vi "Write Waveform to Log File Instance.vi"(6 "Data":dbl[](array[numeric]), 7 "Segmented Log Waveform Meta Data":T1, 8 "error in (no error)":errorcluster, 9 "Channel Name in":string, 11 "Segmented Log in":refnum<class "Segmented Log.lvclass">) -> (0 "error out":errorcluster, 1 "File Segmented":bool, 2 "Log Active":bool, 3 "Segmented Log out":refnum<class "Segmented Log.lvclass">)   [LabVIEW 2012, in "Waveform Data Logger Engine.lvlib" / "Segmented Log.lvclass"]
doc: "Writes data to a log file instance. If the segmented log is still active, ensures a valid file instance is open before logging data. After each write operation, checks if the current file instance has surpassed any limits and needs to be closed."
uses:
  Segmented Log.lvclass
  Segmented Log Waveform Meta Data.ctl
  Segmented Log.lvclass/Segmented Log.ctl
  Shared/Classes/Log File Specifications/Log File Specification/Log File Specification.lvclass/Log File Specification.ctl
  Shared/Classes/Log File Specifications/Waveform TDMS Log File Specification/Waveform TDMS Log File Specification.lvclass
  Shared/Classes/Log File Specifications/Waveform TDMS Log File Specification/Waveform TDMS Log File Specification.lvclass/Waveform TDMS Log File Specification.ctl
  Log Files/Log File/Log File.lvclass/Log File.ctl
  Log Files/TDMS Log File/TDMS Log File.lvclass
  Log Files/TDMS Log File/TDMS Log File.lvclass/TDMS Log File.ctl
  Close Log File Instance.vi
  Open Log File Instance.vi
  On Segmented Log Complete.vi
  On File Close.vi
  Shared/Classes/Log File Specifications/Log File Specification/Open Log File.vi
  Shared/Classes/Log File Specifications/Log File Specification/Set Path Tag.vi
  On File Open.vi
  Shared/Classes/Log File Specifications/Log File Specification/Set Filename Offset.vi
  Shared/Classes/Log File Specifications/Log File Specification/Build File Path.vi
  Shared/Classes/Log File Specifications/Log File Specification/Resolve File Conflicts.vi
  Shared/Classes/Log File Specifications/Log File Specification/Initialize Log File.vi
  <vilib>/Utility/libraryn.llb/Check if File or Folder Exists.vi
  <vilib>/Utility/error.llb/Error Cluster From Error Code.vi
  <vilib>/Utility/libraryn.llb/Get File Extension.vi
  <vilib>/Utility/libraryn.llb/Create Directory Recursive.vi
  Segment Log File.vi
  Log Files/Log File/Close Log File.vi
  Make File Read-Only.vi
  Log Files/Log File/Log File.lvclass
  Shared/Classes/Log File Specifications/Log File Specification/Log File Specification.lvclass
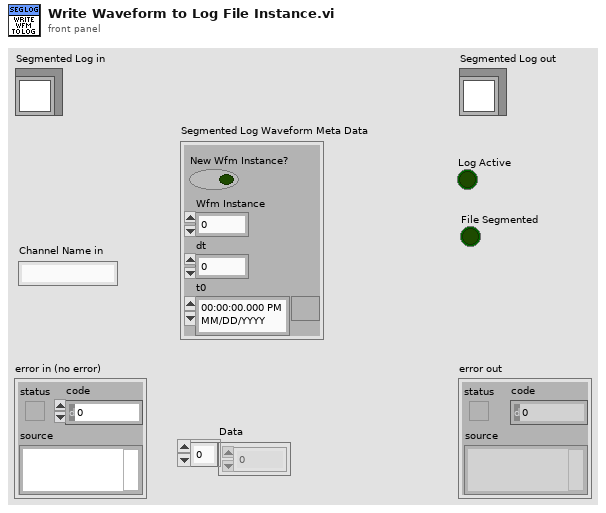
[diagram p1: front panel]
types:
  T1 = typedef "Waveform Data Logger Engine.lvlib/Segmented Log.lvclass/Segmented Log Waveform Meta Data.ctl" = cluster{"New Wfm Instance?":bool, "Wfm Instance":i32, "dt":dbl, "t0":timestamp}
  T2 = typedef "Waveform Data Logger Shared.lvlib/Log File Specification.lvclass/Log Specification Type.ctl" = enum16{"Default", "TDMS", "Text", "Waveform TDMS"}
  T3 = typedef "Waveform Data Logger Engine.lvlib/Log File.lvclass/Log File Type.ctl" = enum16{"Default", "TDMS", "Text"}
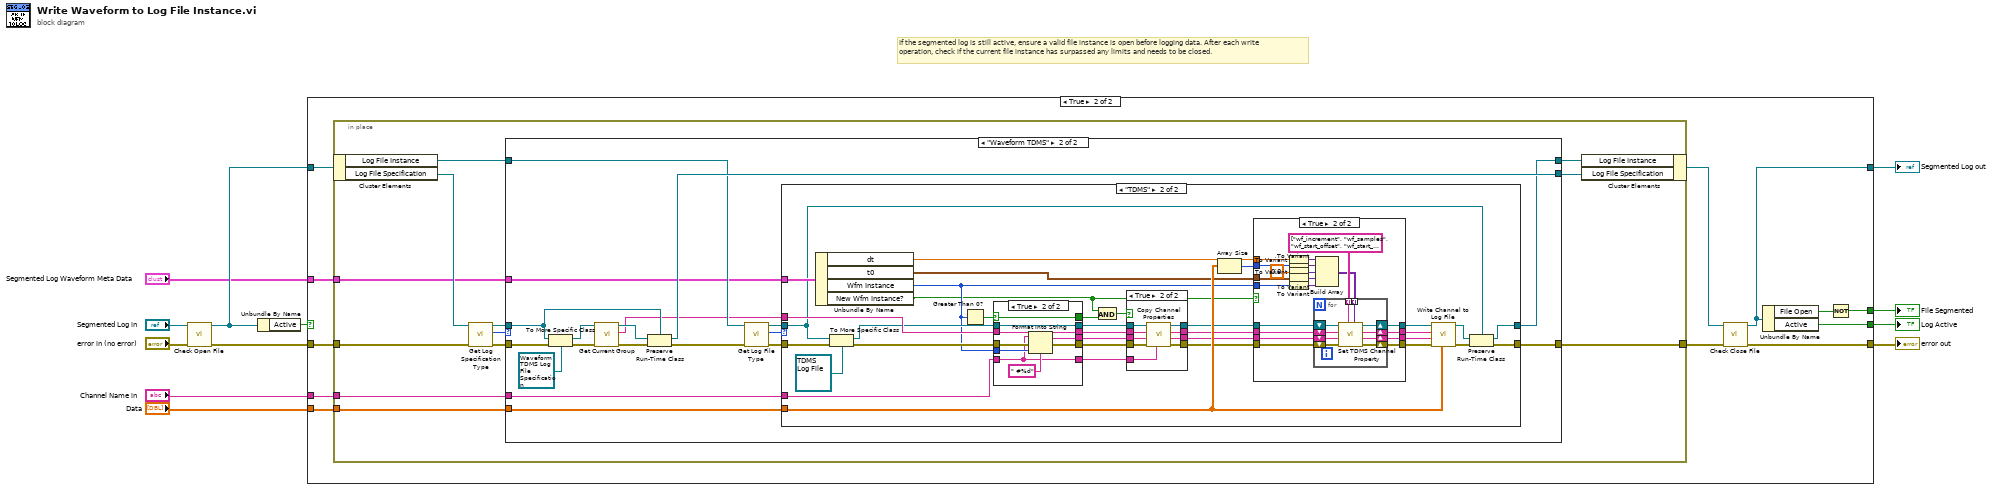
[diagram p0: block diagram]
diagram:
  # "If the segmented log is still active, ensure a valid file instance is open before logging data. After each write operation, check if the current file instance has surpassed any limits and needs to be closed."
  n1 = call "Check Open File.vi"("error in (no error)"="error in (no error)", "Segmented Log in"="Segmented Log in") -> ("error out"=w7:errorcluster, "Segmented Log out"=w6:refnum<class "Segmented Log.lvclass">)  [unwired: 8 in]
  n2 = Unbundle By Name(w6) -> ("Active"=w5:bool)
  n3 = case shown="True" w5 {
    selector: w5 -> [w14 _]
    tunnel: w7 -> [w15 w24]
    tunnel: "Channel Name in" -> [_ w23]
    tunnel: "Data" -> [_ w27]
    tunnel: [w13 w21] -> w10
    tunnel: [w15 w25] -> w11
    tunnel: w6 -> [w13 w22]
    tunnel: [w14 w20] -> w8
    tunnel: "Segmented Log Waveform Meta Data" -> [_ w19]
    tunnel: [_ w16] -> w1
    frame False {
      # "This segmented logging configuration is no longer active."
    }
    frame True {
      n4 = in-place {
        in-place-border: w27 -> [w39]
        in-place-border: [w38] -> w26
        in-place-border: w24 -> [w34]
        in-place-border: w23 -> [w37]
        in-place-border: w19 -> [w29]
        n5 = in-place-cluster #1(w22) -> ("Log File Instance"=w28:refnum<class "Log File.lvclass">, "Log File Specification"=w32:refnum<class "Log File Specification.lvclass">)
        n6 = call "Get Log Specification Type.vi"("error in (no error)"=w34, "Log File Specification in"=w32) -> ("error out"=w33:errorcluster, "Log Specification Type"=w30:T2, "Log File Specification out"=w31:refnum<class "Log File Specification.lvclass">)  [unwired: 7 in]
        n7 = case shown="\"Waveform TDMS\"" w30 {
          tunnel: w39 -> [_ w61]
          tunnel: [w42 w47] -> w38
          tunnel: w37 -> [_ w60]
          tunnel: w28 -> [w41 w51]
          tunnel: [w41 w46] -> w36
          tunnel: [w40 w54] -> w35
          tunnel: w33 -> [w42 w53]
          tunnel: w31 -> [w40 w52]
          tunnel: w29 -> [_ w43]
          frame Default {
            # "TODO-LATER: Throw Error"
          }
          frame "Waveform TDMS" {
            n8 = To More Specific Class(target class=refnum<class "Waveform TDMS Log File Specification.lvclass"> refnum ("Waveform Data Logger Engine.lvlib:Waveform TDMS Log File Specification.lvclass"), reference=w52, error in=w53) -> (specific class reference=w57:refnum<class "Waveform TDMS Log File Specification.lvclass">, error out=w58:errorcluster)
            n9 = call "Get Current Group.vi"("error in (no error)"=w58, "Waveform TDMS Log File Specification in"=w57) -> ("error out"=w56:errorcluster, "Current Group"=w44:string, "Waveform TDMS Log File Specification out"=w55:refnum<class "Waveform TDMS Log File Specification.lvclass">)  [unwired: 7 in]
            n10 = Preserve Run-Time Class(object in=w55, error in=w56, 2:w52) -> (object out=w54:refnum<class "Log File Specification.lvclass">, error out=w50:errorcluster)
            n11 = call "Get Log File Type.vi"("error in (no error)"=w50, "Log File in"=w51) -> ("error out"=w48:errorcluster, "Log File Type"=w45:T3, "Log File out"=w49:refnum<class "Log File.lvclass">)  [unwired: 7 in]
            n12 = case shown="\"TDMS\"" w45 {
              tunnel: w61 -> [_ w82]
              tunnel: w60 -> [_ w77]
              tunnel: w49 -> [w62 w83]
              tunnel: w48 -> [w63 w93]
              tunnel: [w63 w95] -> w47
              tunnel: [w62 w94] -> w46
              tunnel: w44 -> [_ w89]
              tunnel: w43 -> [_ w91]
              frame "Default", Default {
                # "TODO-LATER: Throw error"
                # ": Throw Error"
              }
              frame "TDMS" {
                n13 = Unbundle By Name(w91) -> ("dt"=w87:dbl, "t0"=w64:timestamp, "Wfm Instance"=w80:i32, "New Wfm Instance?"=w65:bool)
                n14 = To More Specific Class(target class=refnum<class "TDMS Log File.lvclass"> refnum ("TDMS Log File in"), reference=w83, error in=w93) -> (specific class reference=w88:refnum<class "TDMS Log File.lvclass">, error out=w90:errorcluster)
                n15 = Greater Than 0?(x=w80) -> (x > 0?=w78:bool)
                n16 = case shown="True" w78 {
                  selector: w78 -> [w145 w150]
                  tunnel: w90 -> [w147 w156]
                  tunnel: w89 -> [w148 w154]
                  tunnel: w77 -> [w146 w151]
                  tunnel: w80 -> [_ w158]
                  tunnel: [w148 w154] -> w72
                  tunnel: [w146 w152] -> w71
                  tunnel: [w147 w153] -> w70
                  tunnel: [w149 w155] -> w73
                  tunnel: w88 -> [w149 w155]
                  tunnel: [w146 w151] -> w76
                  tunnel: [w145 w150] -> w75
                  frame False {
                  }
                  frame True {
                    n17 = Format Into String(format string=" #%d", initial string=w151, error in=w156, w158) -> (resulting string=w152:string, error out=w153:errorcluster)
                  }
                }
                n18 = And(x=w65, y=w75) -> (x .and. y?=w74:bool)
                n19 = case shown="True" w74 {
                  tunnel: w76 -> [_ w110]
                  tunnel: w73 -> [w101 w109]
                  tunnel: w72 -> [w100 w108]
                  tunnel: w71 -> [w99 w107]
                  tunnel: w70 -> [w98 w106]
                  tunnel: [w101 w105] -> w69
                  tunnel: [w100 w104] -> w68
                  tunnel: [w99 w103] -> w67
                  tunnel: [w98 w102] -> w66
                  frame False {
                  }
                  frame True {
                    n20 = call "Copy Channel Properties.vi"("Base Channel"=w110, "error in (no error)"=w106, "New Channel in"=w107, "Group Name in"=w108, "TDMS Log File in"=w109) -> ("error out"=w102:errorcluster, "New Channel out"=w103:string, "Group Name out"=w104:string, "TDMS Log File out"=w105:refnum<class "TDMS Log File.lvclass">)  [unwired: 3 in]
                  }
                }
                n21 = Array Size(array=w82) -> (size(s)=w81:i32)
                n22 = case shown="True" w65 {
                  tunnel: w66 -> [w111 w115]
                  tunnel: w67 -> [w112 w116]
                  tunnel: w68 -> [w113 w117]
                  tunnel: w69 -> [w114 w118]
                  tunnel: w87 -> [_ w120]
                  tunnel: w64 -> [_ w133]
                  tunnel: [w114 w126] -> w86
                  tunnel: [w113 w125] -> w85
                  tunnel: [w112 w124] -> w79
                  tunnel: [w111 w123] -> w84
                  tunnel: w81 -> [_ w122]
                  tunnel: w80 -> [_ w119]
                  frame False {
                  }
                  frame True {
                    n23 = To Variant(anything=w120) -> (Variant=w130:variant)
                    n24 = To Variant(anything=w122) -> (Variant=w128:variant)
                    n25 = To Variant(anything=0.0) -> (Variant=w131:variant)
                    n26 = To Variant(anything=w133) -> (Variant=w129:variant)
                    n27 = To Variant(anything=w119) -> (Variant=w121:variant)
                    n28 = Build Array(w130, w128, w131, w129, w121) -> (w127:variant[])
                    n29 = for {
                      shift-right: [w143] -> w123
                      shift-left: w115 -> [w144]
                      shift-right: [w139] -> w124
                      shift-left: w116 -> [w142]
                      shift-right: [w140] -> w125
                      shift-left: w117 -> [w141]
                      shift-right: [w137] -> w126
                      shift-left: w118 -> [w138]
                      tunnel: string[] ["wf_increment", "wf_samples", "wf_start_offset", "wf_start_time", "Waveform Instance"] ("property names") -> [w136] mode=indexing
                      tunnel: w127 -> [w135] mode=indexing
                      n30 = call "Set TDMS Channel Property.vi"("Property Value"=w135, "Property Name"=w136, "error in (no error)"=w144, "Channel Name in"=w142, "Group Name in"=w141, "TDMS Log File in"=w138) -> ("error out"=w143:errorcluster, "Channel Name out"=w139:string, "Group Name out"=w140:string, "TDMS Log File out"=w137:refnum<class "TDMS Log File.lvclass">)  [unwired: 2 in]
                    }
                  }
                }
                n31 = call "Write Channel to Log File.vi"("Data"=w82, "error in (no error)"=w84, "Channel Name in"=w79, "Group Name in"=w85, "Log File in"=w86) -> ("error out"=w97:errorcluster, "Log File out"=w96:refnum<class "TDMS Log File.lvclass">)  [unwired: 5 in]
                n32 = Preserve Run-Time Class(object in=w96, error in=w97, 2:w83) -> (object out=w94:refnum<class "Log File.lvclass">, error out=w95:errorcluster)
              }
            }
          }
        }
        n33 = in-place-cluster #1("Log File Instance"=w36, "Log File Specification"=w35) -> (w18:refnum<class "Segmented Log.lvclass">)
      }
      n34 = call "Check Close File.vi"("error in (no error)"=w26, "Segmented Log in"=w18) -> ("error out"=w25:errorcluster, "Segmented Log out"=w21:refnum<class "Segmented Log.lvclass">)  [unwired: 8 in]
      n35 = Unbundle By Name(w21) -> ("File Open"=w17:bool, "Active"=w20:bool)
      n36 = Not(x=w17) -> (.not. x?=w16:bool)
    }
  }
  "error out" <- w11
  "Segmented Log out" <- w10
  "Log Active" <- w8
  "File Segmented" <- w1
